vi "Destroy to Session.vi"(8 "Error In":errorcluster, 11 "SFTP":refnum<class "SFTP.lvclass">) -> (0 "Error Out":errorcluster, 3 "Session":refnum<class "Session.lvclass">)   [LabVIEW 2018, in "Toolkit.lvlib" / "SFTP.lvclass"]
doc: "Destroys a SFTP object and returns the Session used to create it. This should be called when interaction with the remote SFTP server is completed. When called, no other VIs in the SFTP class should be called."
uses:
  SFTP.lvclass
  Session/Session.lvclass
  SFTP.lvclass/SFTP.ctl
  Session/Session.lvclass/Session.ctl
  SSH/SSH.lvclass/SSH.ctl
  Toolkit.lvlib
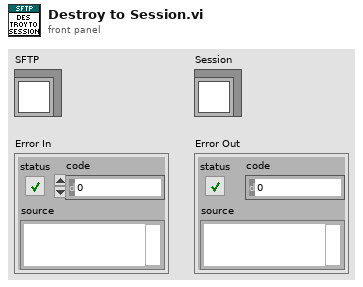
[diagram p1: front panel]
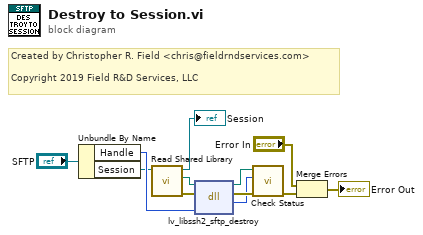
[diagram p0: block diagram]
diagram:
  # "Created by Christopher R. Field <chris@fieldrndservices.com>\n\nCopyright 2019 Field R&D Services, LLC"
  n1 = Unbundle By Name("SFTP") -> ("Handle"=w10:u64, "Session"=w4:refnum<class "Session.lvclass">)
  n2 = call "Read Shared Library.vi"("Session In"=w4) -> ("Erorr Out"=w1:errorcluster, "libssh2lv Shared Library"=w2:path, "Session Out"=→"Session":refnum<class "Session.lvclass">)  [unwired: 8 in]
  n3 = dll-call lib="D:/Users/cfield/Code/Field R&D Services/SSH/LV-LIBSSH2/LabVIEW/trunk/src/Toolkit/Support/lv-libssh2.dll" fn="lv_libssh2_sftp_destroy"(path in=w2, error in=w1, "handle"=w10) -> (path out=w8:path, error out=w9:errorcluster, "status"=w6:i32)  [unwired: 2 in]
  n4 = call "Check Status.vi"("Error In"=w9, "Status"=w6, "libssh2lv Shared Library In"=w8) -> ("Error Out"=w7:errorcluster)  [unwired: 7 in, 1 out]
  n5 = Merge Errors("Error In", w7) -> (→"Error Out":errorcluster)
